vi "Test Generated Voltage Ramp Start at Min Voltage.vi"(8 "error in (no error)":errorcluster, 11 "Ramp Voltage Test In":refnum<class "Ramp Voltage Test.lvclass">) -> (0 "error out":errorcluster, 3 "Ramp Voltage Test Out":refnum<class "Ramp Voltage Test.lvclass">)   [LabVIEW 2020, in "High Level PSU With Tests.lvlib" / "Ramp Voltage Test.lvclass"]
uses:
  Ramp Voltage Test.lvclass
  C:/Program Files (x86)/National Instruments/LabVIEW 2020/vi.lib/Astemes/LUnit/Test Case.lvclass
  Ramp Voltage/Ramp Settings.ctl
  Ramp Voltage/Ramp Voltage.lvclass
  Mock Voltage Output/Mock Voltage Output.lvclass
  C:/Git/astemes-gdevcon-2022/PSU Demo/High Level PSU With Tests/Voltage Output/Voltage Output.lvclass
  Ramp Voltage/Ramp Voltage.lvclass/Ramp Voltage.ctl
  <vilib>/Astemes/LUnit/Test Case.lvclass/Test Case.ctl
  01074fa8-ee8a-411d-bc8b-fc92c4f90959.vi
  <vilib>/Astemes/LUnit/Palette/Pass.vi
  <vilib>/Astemes/LUnit/Palette/Fail.vi
  <vilib>/Astemes/LUnit/Compare Variants.vi
  <vilib>/Astemes/LUnit/Describe Comparison.vi
  <vilib>/Astemes/LUnit/Set Assertion Type.vi
  <vilib>/Astemes/LUnit/Add test result.vi
  <vilib>/Astemes/LUnit/Variant to string.vi
  <vilib>/Astemes/LUnit/LUnit Record Assertion Result.vi
  <vilib>/Astemes/LUnit/LUnit Aggregate Assertion Results.vi
  <vilib>/Astemes/LUnit/Method Result/LUnit Merge Status.vi
  <vilib>/Astemes/LUnit/LUnit Concatenate result strings.vi
  <vilib>/Utility/Data Type/Get Type Information.vi
  <vilib>/Utility/LVClass/Get LV Class Name.vi
  Ramp Voltage Test.lvclass/Ramp Voltage Test.ctl
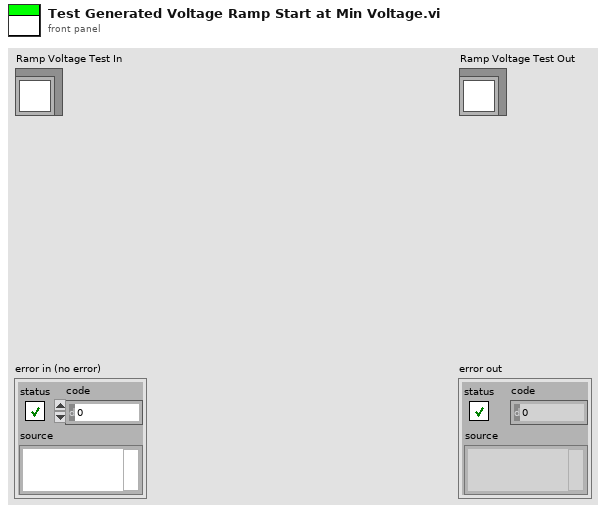
[diagram p1: front panel]
types:
  T1 = typedef "High Level PSU With Tests.lvlib/Ramp Voltage.lvclass/Ramp Settings.ctl" = cluster{"Max Output Voltage [V]":dbl, "Min Output Voltage [V]":dbl, "Step Size [V]":dbl, "Ramp Time [s]":dbl}
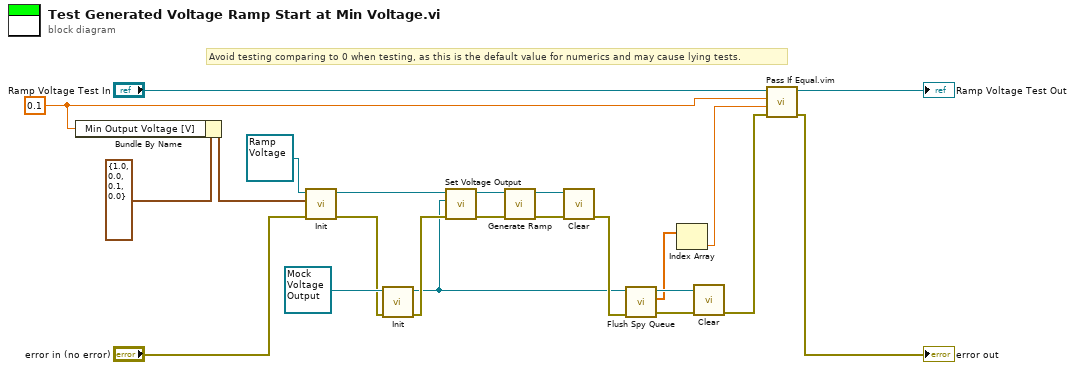
[diagram p0: block diagram]
diagram:
  w1 = 0.1 ("Min Output Voltage [V]")
  # "Avoid testing comparing to 0 when testing, as this is the default value for numerics and may cause lying tests."
  n1 = Bundle By Name(cluster=T1 {"Max Output Voltage [V]"=1.0, "Min Output Voltage [V]"=0.0, "Step Size [V]"=0.1, "Ramp Time [s]"=0.0} ("Settings"), "Min Output Voltage [V]"=w1) -> (w2:T1)
  n2 = call "Init.vi"("error in (no error)"="error in (no error)", "Settings"=w2, "Ramp Voltage In"=refnum<class "Ramp Voltage.lvclass"> refnum ("Ramp Use Case In")) -> ("error out"=w16:errorcluster, "Ramp Voltage Out"=w20:refnum<class "Ramp Voltage.lvclass">)  [unwired: 7 in]
  n3 = call "Init.vi"("error in (no error)"=w16, "Mock Voltage Output In"=refnum<class "Mock Voltage Output.lvclass"> refnum) -> ("error out"=w15:errorcluster, "Mock Voltage Output Out"=w6:refnum<class "Mock Voltage Output.lvclass">)  [unwired: 8 in]
  n4 = call "Set Voltage Output.vi"("error in (no error)"=w15, "Voltage Output"=w6, "Ramp Voltage In"=w20) -> ("error out"=w14:errorcluster, "Ramp Voltage Out"=w4:refnum<class "Ramp Voltage.lvclass">)  [unwired: 7 in]
  n5 = call "Generate Ramp.vi"("error in (no error)"=w14, "Ramp Use Case In"=w4) -> ("error out"=w5:errorcluster, "Ramp Use Case Out"=w3:refnum<class "Ramp Voltage.lvclass">)  [unwired: 8 in]
  n6 = call "Clear.vi"("error in (no error)"=w5, "Ramp Use Case in"=w3) -> ("error out"=w10:errorcluster)  [unwired: 8 in, 1 out]
  n7 = call "Flush Spy Queue.vi"("error in (no error)"=w10, "Mock Voltage Output in"=w6) -> ("error out"=w11:errorcluster, "Setpoints"=w8:dbl[], "Mock Voltage Output out"=w9:refnum<class "Mock Voltage Output.lvclass">)  [unwired: 7 in]
  n8 = Index Array(array=w8) -> (element=w7:dbl)  [unwired: 1 in]
  n9 = call "Clear.vi"("error in (no error)"=w11, "Mock Voltage Output In"=w9) -> ("error out"=w12:errorcluster)  [unwired: 8 in, 1 out]
  n10 = call "Pass If Equal.vim"("error in (no error)"=w12, "Actual"=w7, "Expected"=w1, "LUnit Test Case In"="Ramp Voltage Test In") -> ("error out"=→"error out":errorcluster, "LUnit Test Case Out"=→"Ramp Voltage Test Out":refnum<class "Ramp Voltage Test.lvclass">)  [unwired: 6 in]
